vi "Thorlabs_CageRotator_ActiveX_Full.vi"(8 "error in (no error)":errorcluster, 11 "HWSerialNum":i32=27264338) -> (0 "error out":errorcluster)   [LabVIEW 2022 SP3]
panel:
  out "Current position":sgl
  in  "Jog (°)":sgl=5.0 min=0 max=360 step=1
  in  "Move +":bool
  in  "Move -":bool
  in  "Move absolute (°)":dbl min=0.0 max=360.0 step=1.0
  in  "Home Button":bool
  in  "stop":bool
  in  "MG17Motor":refnum<k7>(container)
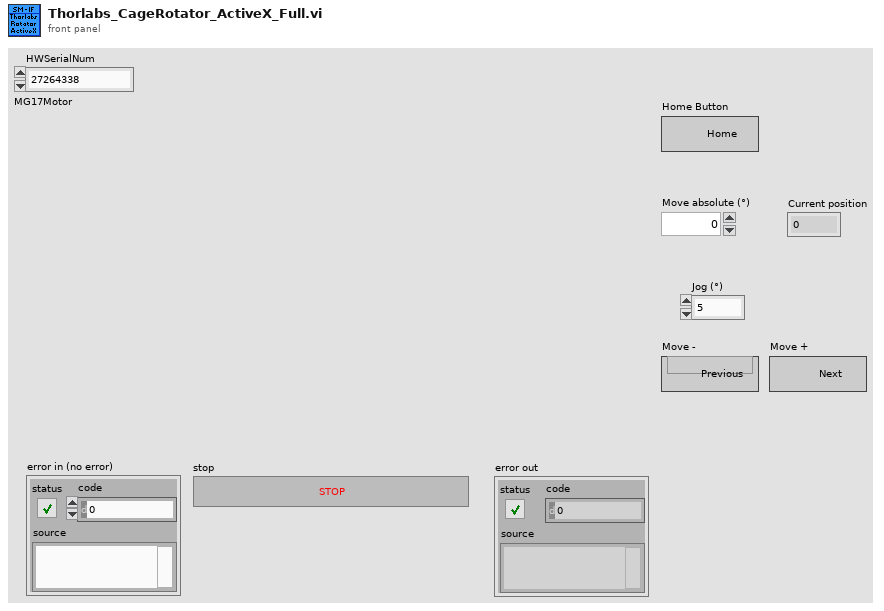
[diagram p1: front panel]
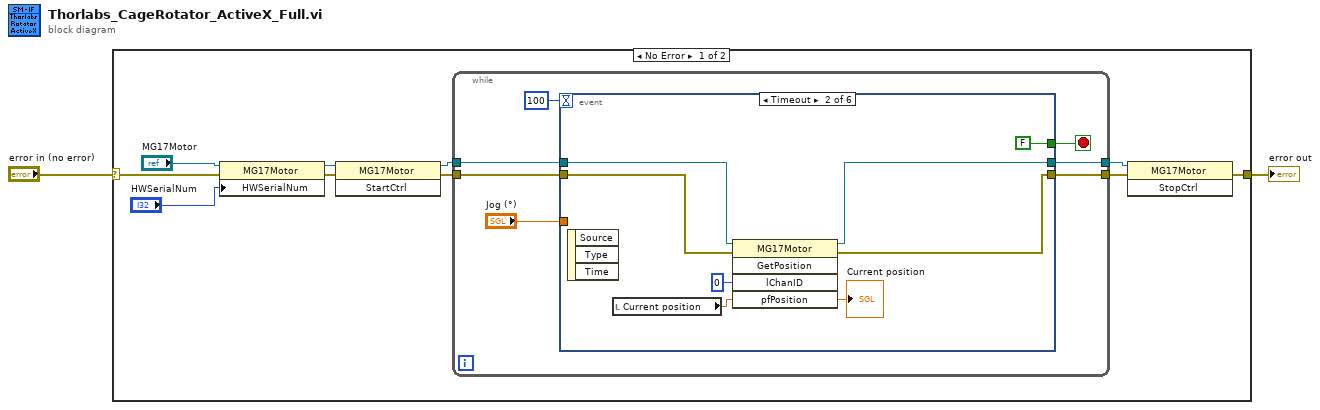
[diagram p0: block diagram]
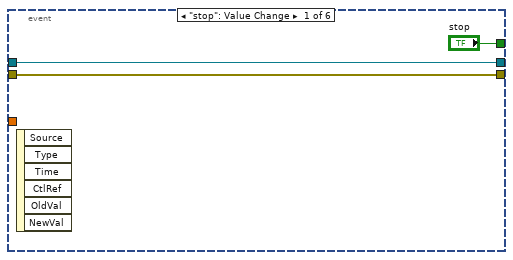
[diagram p2: hidden frame]
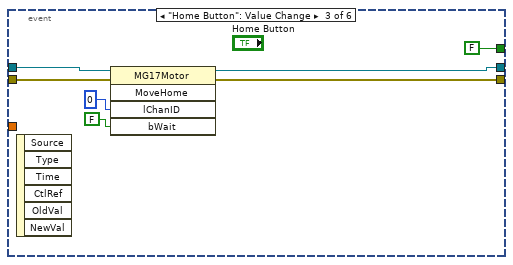
[diagram p3: hidden frame]
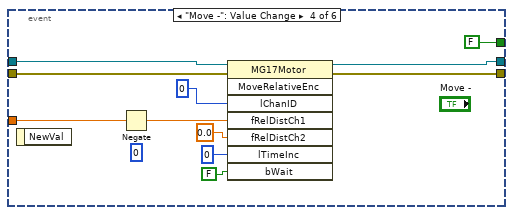
[diagram p4: hidden frame]
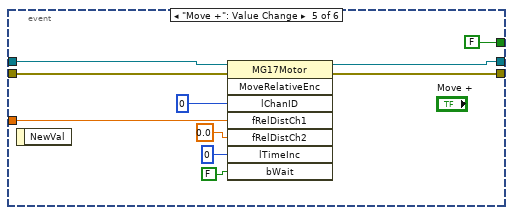
[diagram p5: hidden frame]
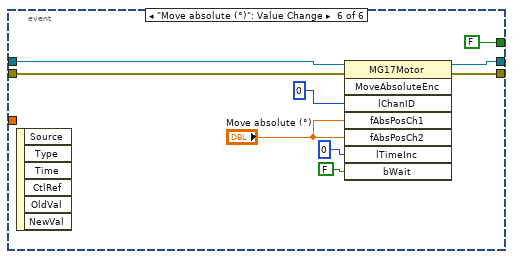
[diagram p6: hidden frame]
diagram:
  n1 = case shown="No Error" "error in (no error)" {
    selector: "error in (no error)" -> [w3 w68]
    tunnel: [w4 w68] -> w2
    frame No Error {
      n2 = property class="MG17Motor"(reference="MG17Motor", error in=w3, "HWSerialNum"="HWSerialNum") -> (reference out=w10:refnum<k7>, error out=w9:errorcluster)
      n3 = invoke class="MG17Motor" method="StartCtrl"(reference=w10, error in=w9) -> (reference out=w7:refnum<k7>, error out=w5:errorcluster)  [unwired: 1 in, 1 out]
      n4 = while {
        tunnel: [w14] -> w8
        tunnel: w7 -> [w17]
        tunnel: [w16] -> w6
        tunnel: w5 -> [w15]
        stop <- w18 stop-if-true
        n5 = event shown="[1] Timeout" {
          selector: _ -> [_ _ _ _ _ _]
          dyn-events: _ -> [_ _ _ _ _ _]
          timeout: 100 -> [_ _ _ _ _ _]
          tunnel: ["stop" FALSE ("stop") FALSE ("stop") FALSE ("stop") FALSE ("stop") FALSE ("stop")] -> w18
          tunnel: w17 -> [w20 w28 w37 w48 w57 w66]
          tunnel: w15 -> [w21 w29 w36 w47 w56 w65]
          tunnel: [w21 w26 w35 w46 w50 w63] -> w16
          tunnel: [w20 w27 w32 w45 w51 w64] -> w14
          tunnel: "Jog (°)" -> [_ _ _ w40 w55 _]
          event "stop": Value Change {
            n6 = event-data() -> ()  [unwired: 1 in, 6 out]
          }
          event Timeout {
            n7 = event-data() -> ()  [unwired: 1 in, 3 out]
            n8 = local read "Current position"() -> (w23:sgl)
            n9 = invoke class="MG17Motor" method="GetPosition"(reference=w28, error in=w29, "lChanID"=0, "pfPosition"=w23) -> (reference out=w27:refnum<k7>, error out=w26:errorcluster, "pfPosition"=→"Current position":sgl)  [unwired: 1 in, 2 out]
          }
          event "Home Button": Value Change {
            n10 = event-data() -> ()  [unwired: 1 in, 6 out]
            n11 = invoke class="MG17Motor" method="MoveHome"(reference=w37, error in=w36, "lChanID"=0, "bWait"=FALSE) -> (reference out=w32:refnum<k7>, error out=w35:errorcluster)  [unwired: 1 in, 3 out]
          }
          event "Move -": Value Change {
            (unwired) 0 ("lJogDir")
            n12 = event-data() -> ()  [unwired: 1 in, 1 out]
            n13 = Negate(x=w40) -> (-x=w38:sgl)
            n14 = invoke class="MG17Motor" method="MoveRelativeEnc"(reference=w48, error in=w47, "lChanID"=0, "fRelDistCh1"=w38, "fRelDistCh2"=sgl 0.0, "lTimeInc"=0, "bWait"=FALSE) -> (reference out=w45:refnum<k7>, error out=w46:errorcluster)  [unwired: 1 in, 6 out]
          }
          event "Move +": Value Change {
            n15 = event-data() -> ()  [unwired: 1 in, 1 out]
            n16 = invoke class="MG17Motor" method="MoveRelativeEnc"(reference=w57, error in=w56, "lChanID"=0, "fRelDistCh1"=w55, "fRelDistCh2"=sgl 0.0, "lTimeInc"=0, "bWait"=FALSE) -> (reference out=w51:refnum<k7>, error out=w50:errorcluster)  [unwired: 1 in, 6 out]
          }
          event "Move absolute (°)": Value Change {
            n17 = event-data() -> ()  [unwired: 1 in, 6 out]
            n18 = invoke class="MG17Motor" method="MoveAbsoluteEnc"(reference=w66, error in=w65, "lChanID"=0, "fAbsPosCh1"="Move absolute (°)", "fAbsPosCh2"="Move absolute (°)", "lTimeInc"=0, "bWait"=FALSE) -> (reference out=w64:refnum<k7>, error out=w63:errorcluster)  [unwired: 1 in, 6 out]
          }
        }
      }
      n19 = invoke class="MG17Motor" method="StopCtrl"(reference=w8, error in=w6) -> (error out=w4:errorcluster)  [unwired: 1 in, 2 out]
    }
    frame Error {
    }
  }
  "error out" <- w2
